vi "LEDExecute.vi"(8 "error in (no error)":errorcluster) -> (0 "error out":errorcluster)   [LabVIEW 2023]
uses:
  Robot Global Data.vi
  GeneralPurpose/AllianceColorGlobal.vi
  Drive/DriveGlobal.vi
  Intake/IntakeGlobal.vi
  Human/HumanGlobal.vi
  Intake/IntakeStates.ctl
  <vilib>/Rock Robotics/WPI/ThirdParty/PhotonVisionLib/PhotonVisionLib.lvlib
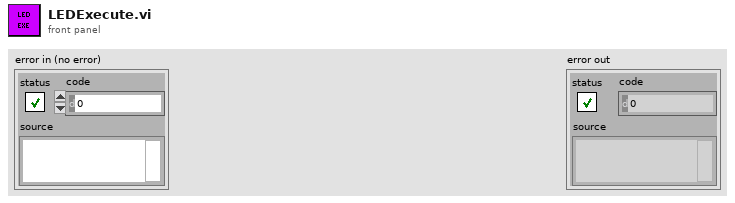
[diagram p1: front panel]
types:
  T1 = typedef "IntakeStates.ctl" = enum16{"Start", "WaitForCommand", "IntakeCoral", "IntakeAlgae", "WaitForCoral", "WaitForAlgae", "DepositCoral", "DepositAlgae", "DepositCoralTimer", "DepositAlgaeTimer"}
  T2 = typedef "WPI_DigitalOutputDevRef.ctl" = cluster{"DIO Channel":T3, "DevStatus":errorcluster}
  T3 = typedef "FPGA_DIOChannel.ctl" = enum8{"DIO 0", "DIO 1", "DIO 2", "DIO 3", "DIO 4", "DIO 5", "DIO 6", "DIO 7", "DIO 8", "DIO 9", "DIO MXP 0", "DIO MXP 1", "DIO MXP 2", "DIO MXP 3", "DIO MXP 4", "DIO MXP 5", "DIO MXP 6", "DIO MXP 7", "DIO MXP 8", "DIO MXP 9", "DIO MXP 10", "DIO MXP 11", "DIO MXP 12", "DIO MXP 13", "DIO MXP 14", "DIO MXP 15", "SPI Port CS1", "SPI Port CS2", "SPI Port CS3", "SPI Port MISO", "SPI Port MOSI", "Invalid"}
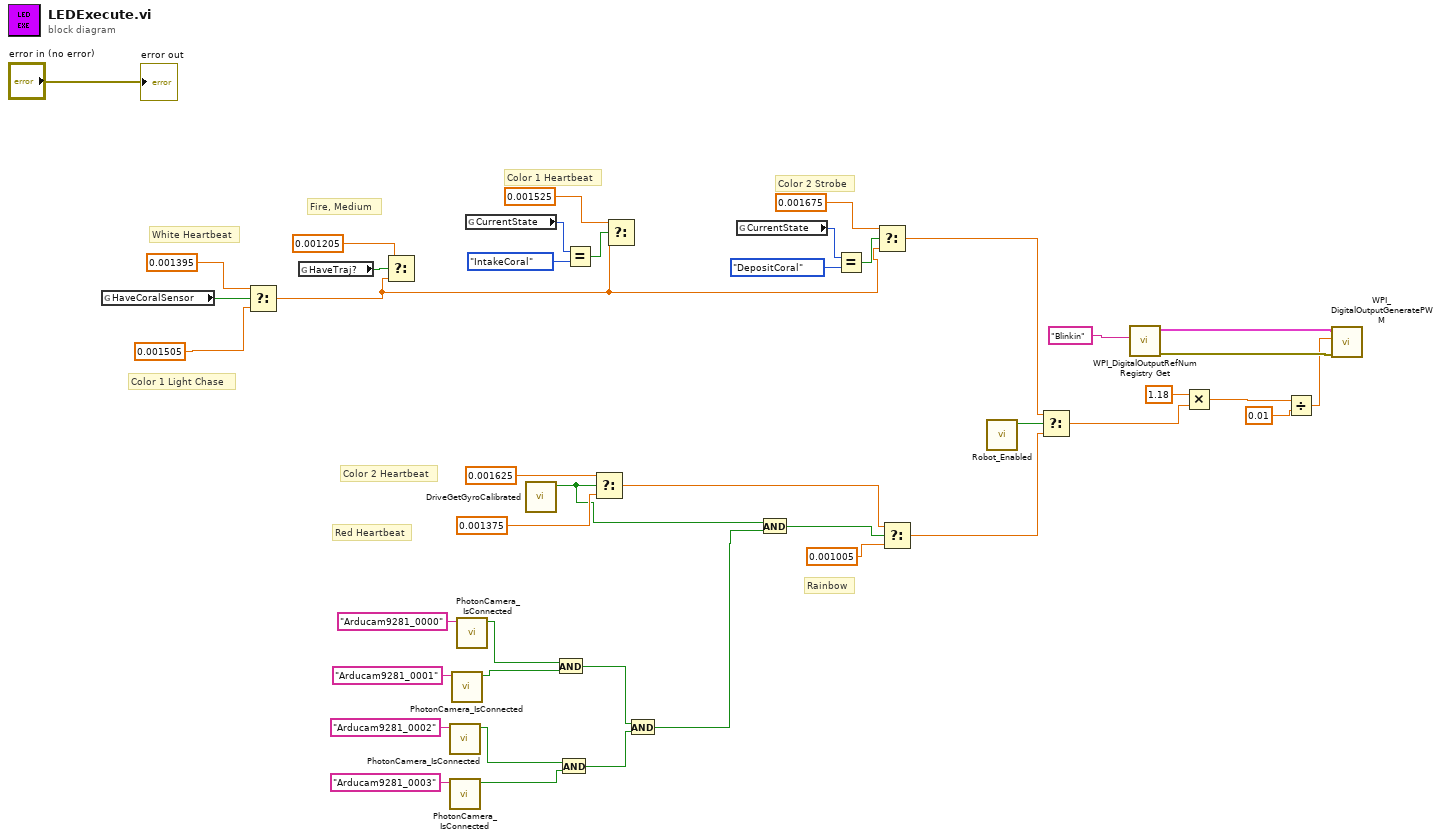
[diagram p0: block diagram]
diagram:
  # "Rainbow"
  # "Color 2 Strobe"
  # "Color 1 Heartbeat"
  # "Color 1 Light Chase"
  # "White Heartbeat"
  # "Fire, Medium"
  # "Color 2 Heartbeat"
  # "Red Heartbeat"
  n1 = global read "IntakeGlobal.vi" "HaveCoralSensor"() -> (w39:bool)
  n2 = Select(t=0.001395, s=w39, f=0.001505 ("t")) -> (s? t:f=w18:dbl)
  n3 = global read "HumanGlobal.vi" "HaveTraj?"() -> (w29:bool)
  n4 = Select(t=0.001205, s=w29, f=w18) -> ()  [unwired: 1 out]
  n5 = call <vilib>:"PhotonCamera_IsConnected.vi"("CameraName"="Arducam9281_0002") -> ("IsConnected"=w10:bool)  [unwired: 9 in, 1 out]
  n6 = call <vilib>:"PhotonCamera_IsConnected.vi"("CameraName"="Arducam9281_0003") -> ("IsConnected"=w9:bool)  [unwired: 9 in, 1 out]
  n7 = call <vilib>:"PhotonCamera_IsConnected.vi"("CameraName"="Arducam9281_0001") -> ("IsConnected"=w11:bool)  [unwired: 9 in, 1 out]
  n8 = call <vilib>:"PhotonCamera_IsConnected.vi"("CameraName"="Arducam9281_0000") -> ("IsConnected"=w12:bool)  [unwired: 9 in, 1 out]
  n9 = global read "IntakeGlobal.vi" "CurrentState"() -> (w25:T1)
  n10 = call "DriveGetGyroCalibrated.vi"() -> ("GryoCalibrated"=w3:bool)  [unwired: 11 in]
  n11 = And(x=w12, y=w11) -> (x .and. y?=w8:bool)
  n12 = And(x=w10, y=w9) -> (x .and. y?=w7:bool)
  n13 = Equal?(x=w25, y=IntakeStates."IntakeCoral") -> (x = y?=w23:bool)
  n14 = Select(t=0.001625, s=w3, f=0.001375 ("t")) -> (s? t:f=w6:dbl)
  n15 = Select(t=0.001525, s=w23, f=w18) -> ()  [unwired: 1 out]
  n16 = And(x=w8, y=w7) -> (x .and. y?=w2:bool)
  n17 = global read "IntakeGlobal.vi" "CurrentState"() -> (w21:T1)
  n18 = And(x=w3, y=w2) -> (x .and. y?=w1:bool)
  n19 = Equal?(x=w21, y=IntakeStates."DepositCoral") -> (x = y?=w19:bool)
  n20 = Select(t=0.001675, s=w19, f=w18) -> (s? t:f=w16:dbl)
  n21 = Select(t=w6, s=w1, f=0.001005) -> (s? t:f=w4:dbl)
  n22 = call "Robot_Enabled.vi"() -> ("Robot Enabled"=w43:bool)  [unwired: 11 in]
  n23 = Select(t=w16, s=w43, f=w4) -> (s? t:f=w31:dbl)
  n24 = call <vilib>:"WPI_DigitalOutputRefNum Registry Get.vi"("refnum name"="Blinkin") -> ("error out"=w36:errorcluster, "DigitalOutputDevRef"=w35:T2)  [unwired: 9 in]
  n25 = Multiply(x=1.18, y=w31) -> (x*y=w32:dbl)
  n26 = Divide(x=w32, y=0.01 ("x")) -> (x/y=w34:dbl)
  n27 = call <vilib>:"WPI_DigitalOutputGeneratePWM.vi"("error in (no error)"=w36, "PWM Duty Cycle"=w34, "DigitalOutputDevRef"=w35) -> ()  [unwired: 7 in, 2 out]
  "error out" <- "error in (no error)"
